vi "initialize.vi"(0 "HGF_GPG":refnum<class "HGF_GPG.lvclass">, 3 "initializationData":variant, 5 "error in (no error)":errorcluster, 7 "binaryString":string, 8 "I8 Array":i8[](array[numeric]), 9 "prependSize? (T)":bool, 11 "byteOrder (0:big-endian, network order)":T1(ring)) -> (14 "dup HGF_GPG":refnum<class "HGF_GPG.lvclass">, 17 "found":bool, 19 "error out":errorcluster)   [LabVIEW 2012, in "HGF_GPG.lvlib" / "HGF_GPG.lvclass"]
doc: "This is a dynamic dispatch VI to be implemented by child classes to initialize their attributes.\n\n<B>Recommendation:</B> Use Variant for initialization data."
uses:
  HGF_GPG.lvclass
  HGF_BaseClasses/HGF_Base/HGF_Base.lvclass
  HGF_GPG.lvclass/HGF_GPG.ctl
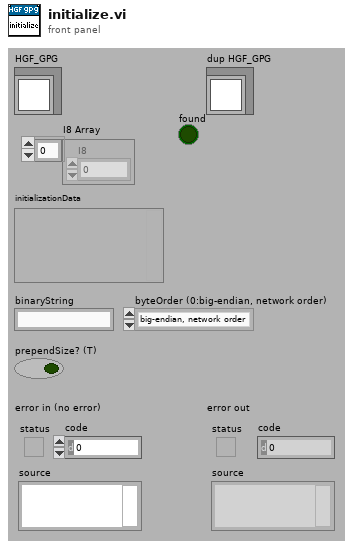
[diagram p1: front panel]
types:
  T1 = enum16{"big-endian, network order", "native, host order", "little-endian"}
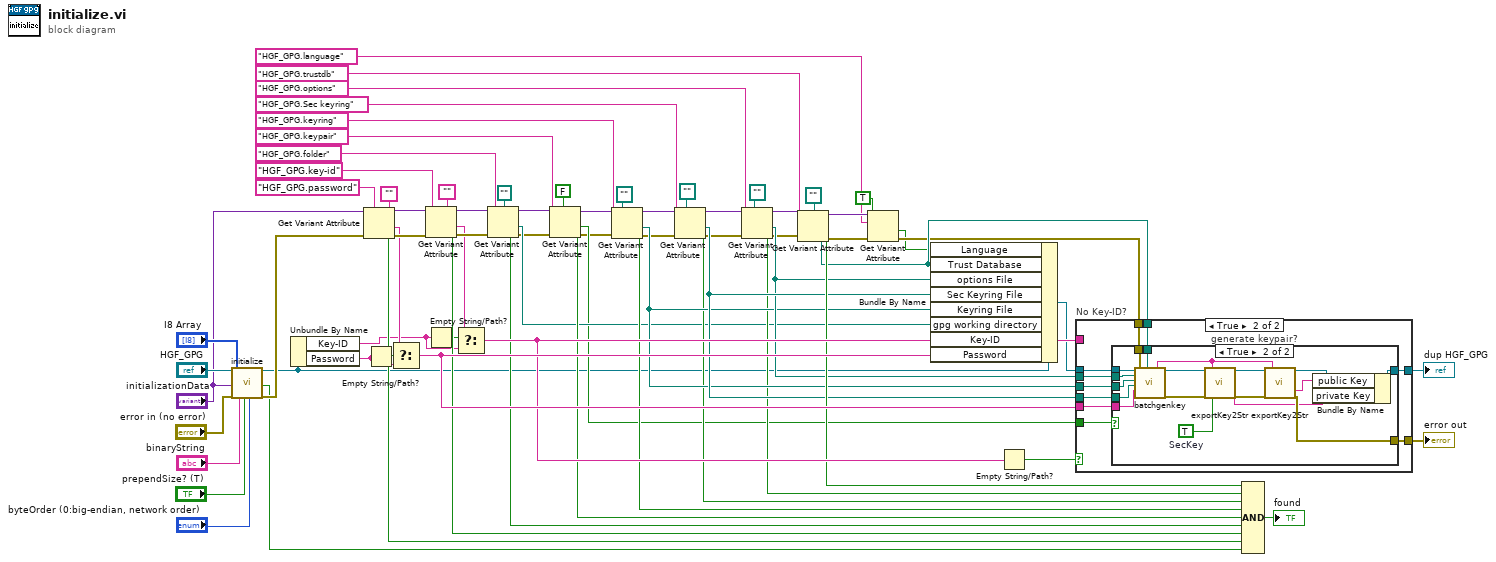
[diagram p0: block diagram]
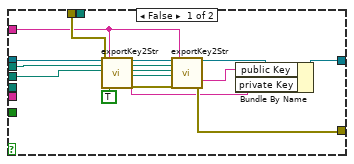
[diagram p2: hidden frame]
diagram:
  n1 = call-parent "initialize.vi"("HGF_Base"="HGF_GPG", "initializationData"="initializationData", "error in (no error)"="error in (no error)", "binaryString"="binaryString", "I8 Array"="I8 Array", "prependSize? (T)"="prependSize? (T)", "byteOrder (0:big-endian, network order)"="byteOrder (0:big-endian, network order)") -> ("dup HGF_Base"=w13:refnum<class "HGF_GPG.lvclass">, "found?"=w40:bool, "error out"=w49:errorcluster)  [unwired: 10 out]
  n2 = Unbundle By Name(w13) -> ("Key-ID"=w8:string, "Password"=w10:string)
  n3 = Get Variant Attribute(Variant="initializationData", name="HGF_GPG.password", default value (empty Variant)="", error in=w49) -> (duplicate Variant=w50:variant, found=w45:bool, value=w12:string, error out=w62:errorcluster)
  n4 = Empty String/Path?(string/path=w10) -> (empty?=w11:bool)
  n5 = Select(t=w12, s=w11, f=w10) -> (s? t:f=w73:string)
  n6 = Get Variant Attribute(Variant=w50, name="HGF_GPG.key-id", default value (empty Variant)="", error in=w62) -> (duplicate Variant=w46:variant, found=w44:bool, value=w7:string, error out=w48:errorcluster)
  n7 = Empty String/Path?(string/path=w8) -> (empty?=w9:bool)
  n8 = Select(t=w7, s=w9, f=w8) -> (s? t:f=w72:string)
  n9 = Get Variant Attribute(Variant=w46, name="HGF_GPG.folder", default value (empty Variant)=path "", error in=w48) -> (duplicate Variant=w38:variant, found=w67:bool, value=w42:path, error out=w37:errorcluster)
  n10 = Get Variant Attribute(Variant=w38, name="HGF_GPG.keypair", default value (empty Variant)=FALSE, error in=w37) -> (duplicate Variant=w30:variant, found=w66:bool, value=w34:bool, error out=w29:errorcluster)
  n11 = Get Variant Attribute(Variant=w30, name="HGF_GPG.keyring", default value (empty Variant)=path "", error in=w29) -> (duplicate Variant=w24:variant, found=w65:bool, value=w68:path, error out=w22:errorcluster)
  n12 = Get Variant Attribute(Variant=w24, name="HGF_GPG.Sec keyring", default value (empty Variant)=path "", error in=w22) -> (duplicate Variant=w23:variant, found=w63:bool, value=w70:path, error out=w21:errorcluster)
  n13 = Get Variant Attribute(Variant=w23, name="HGF_GPG.options", default value (empty Variant)=path "", error in=w21) -> (duplicate Variant=w15:variant, found=w64:bool, value=w69:path, error out=w18:errorcluster)
  n14 = Get Variant Attribute(Variant=w15, name="HGF_GPG.trustdb", default value (empty Variant)=path "", error in=w18) -> (duplicate Variant=w4:variant, found=w71:bool, value=w14:path, error out=w6:errorcluster)
  n15 = Get Variant Attribute(Variant=w4, name="HGF_GPG.language", default value (empty Variant)=TRUE, error in=w6) -> (value=w1:bool, error out=w5:errorcluster)  [unwired: 2 out]
  n16 = Bundle By Name(cluster=w13, "Language"=w1, "Trust Database"=w14, "options File"=w69, "Sec Keyring File"=w70, "Keyring File"=w68, "gpg working directory"=w42, "Key-ID"=w72, "Password"=w73) -> (w33:refnum<class "HGF_GPG.lvclass">)
  n17 = Empty String/Path?(string/path=w72) -> (empty?=w31:bool)
  n18 = case "No Key-ID?" shown="True" w31 {
    tunnel: [w89 w99] -> w32
    tunnel: w5 -> [w87 w97]
    tunnel: [w86 w96] -> w41
    tunnel: w34 -> [_ w98]
    tunnel: w33 -> [w83 w95]
    tunnel: w68 -> [w81 w94]
    tunnel: w69 -> [w82 w93]
    tunnel: w72 -> [w74 _]
    tunnel: w70 -> [_ w92]
    tunnel: w73 -> [_ w91]
    tunnel: w14 -> [_ w90]
    frame False {
      n19 = call-dynamic "exportKey2Str.vi"("HGF_GPG in"=w83, "options file"=w82, "keyringfile"=w81, "error in (no error)"=w87, "key-id"=w74, "SecKey (f)"=TRUE ("SecKey")) -> ("HGF_GPG out"=w85:refnum<class "HGF_GPG.lvclass">, "dup options file"=w77:path, "dup keyringfile"=w78:path, "dup Sec keyringfile"=w79:path, "Key"=w76:string, "error out"=w84:errorcluster)  [unwired: 2 in, 6 out]
      n20 = call-dynamic "exportKey2Str.vi"("HGF_GPG in"=w85, "options file"=w77, "keyringfile"=w78, "Sec keyringfile"=w79, "error in (no error)"=w84, "key-id"=w74) -> ("HGF_GPG out"=w88:refnum<class "HGF_GPG.lvclass">, "Key"=w75:string, "error out"=w86:errorcluster)  [unwired: 2 in, 9 out]
      n21 = Bundle By Name(cluster=w88, "public Key"=w75, "private Key"=w76) -> (w89:refnum<class "HGF_GPG.lvclass">)
    }
    frame True {
      n22 = case "generate keypair?" shown="True" w98 {
        tunnel: w95 -> [w100 w119]
        tunnel: [w100 w113] -> w99
        tunnel: w97 -> [w101 w118]
        tunnel: [w101 w111] -> w96
        tunnel: w94 -> [_ w110]
        tunnel: w93 -> [_ w109]
        tunnel: w92 -> [_ w104]
        tunnel: w91 -> [_ w103]
        tunnel: w90 -> [_ w102]
        frame False {
        }
        frame True {
          w108 = TRUE  # SecKey
          n23 = call-dynamic "batchgenkey.vi"("HGF_GPG in"=w119, "options file"=w109, "keyringfile"=w110, "Sec keyringfile"=w104, "password"=w103, "error in (no error)"=w118, "Trust DB"=w102) -> ("Key-ID"=w105:string, "HGF_GPG out"=w114:refnum<class "HGF_GPG.lvclass">, "error out"=w112:errorcluster)  [unwired: 1 in, 9 out]
          n24 = call-dynamic "exportKey2Str.vi"("HGF_GPG in"=w114, "error in (no error)"=w112, "key-id"=w105, "SecKey (f)"=w108) -> ("HGF_GPG out"=w116:refnum<class "HGF_GPG.lvclass">, "Key"=w107:string, "error out"=w115:errorcluster)  [unwired: 4 in, 9 out]
          n25 = call-dynamic "exportKey2Str.vi"("HGF_GPG in"=w116, "error in (no error)"=w115, "key-id"=w105) -> ("HGF_GPG out"=w117:refnum<class "HGF_GPG.lvclass">, "Key"=w106:string, "error out"=w111:errorcluster)  [unwired: 5 in, 9 out]
          n26 = Bundle By Name(cluster=w117, "public Key"=w106, "private Key"=w107) -> (w113:refnum<class "HGF_GPG.lvclass">)
        }
      }
    }
  }
  "error out" <- w41
  "dup HGF_GPG" <- w32
  n27 = Compound Arithmetic op=AND(w71, w64, w63, w65, w66, w67, w44, w45, w40) -> (→"found":bool)
